vi "NI clear all tasks.vi"(8 "error in (no error)":errorcluster, 11 "NI in":refnum<class "NI.lvclass">) -> (0 "error out":errorcluster, 3 "NI out":refnum<class "NI.lvclass">)   [LabVIEW 2021, in "NI.lvlib" / "NI.lvclass"]
uses:
  NI.lvclass
  NI.lvclass/NI.ctl
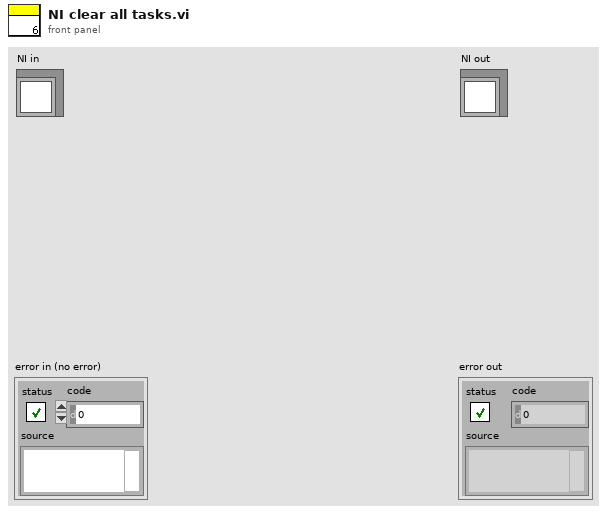
[diagram p1: front panel]
types:
  T1 = cluster{"AO1 laser":refnum<k21>, "AO2 zy":refnum<k21>, "CO1 mainTrig":refnum<k21>, "CO2 fastClock":refnum<k21>, "AI phase":refnum<k21>}
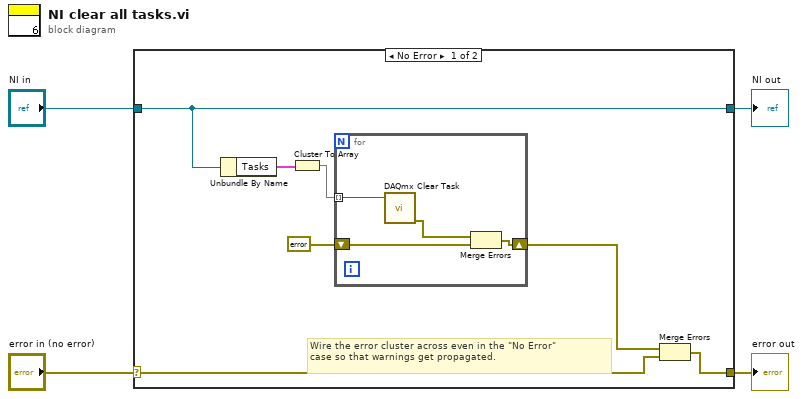
[diagram p0: block diagram]
diagram:
  n1 = case shown="No Error" "error in (no error)" {
    selector: "error in (no error)" -> [w6 w17]
    tunnel: [w5 w17] -> w3
    tunnel: [w11 w16] -> w1
    tunnel: "NI in" -> [w11 w16]
    frame No Error {
      # "Wire the error cluster across even in the \"No Error\"\ncase so that warnings get propagated."
      n2 = Unbundle By Name(w11) -> ("Tasks"=w10:T1)
      n3 = Cluster To Array(cluster=w10) -> (array=w9:refnum<k21>[])
      n4 = for {
        tunnel: w9 -> [w15] mode=indexing
        shift-right: [w12] -> w7
        shift-left: errorcluster {"status"=FALSE, "code"=0, "source"=""} ("error in") -> [w13]
        n5 = call <vilib>:"DAQmx Clear Task.vi"("task in"=w15) -> ("error out"=w14:errorcluster)  [unwired: 14 in]
        n6 = Merge Errors(w14, w13) -> (w12:errorcluster)
      }
      n7 = Merge Errors(w7, w6) -> (w5:errorcluster)
    }
    frame Error {
    }
  }
  "error out" <- w3
  "NI out" <- w1
